vi "MessageTimeOk.vi"(2 "time (ms)":i32=2000, 4 "missage":string) -> ()   [LabVIEW 2015, in "VIPM2.lvlib"]
doc: "Show a message to user in a new window, height dinamicly. Closed by OK button or parametric time (ms)."
uses:
  VIPM2.lvlib
panel:
  in  "Button":bool
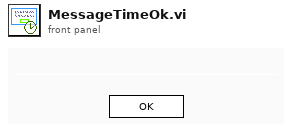
[diagram p1: front panel]
types:
  T1 = typedef "LVRectTypeDef.ctl" = cluster{"Left":i16, "Top":i16, "Right":i16, "Bottom":i16}
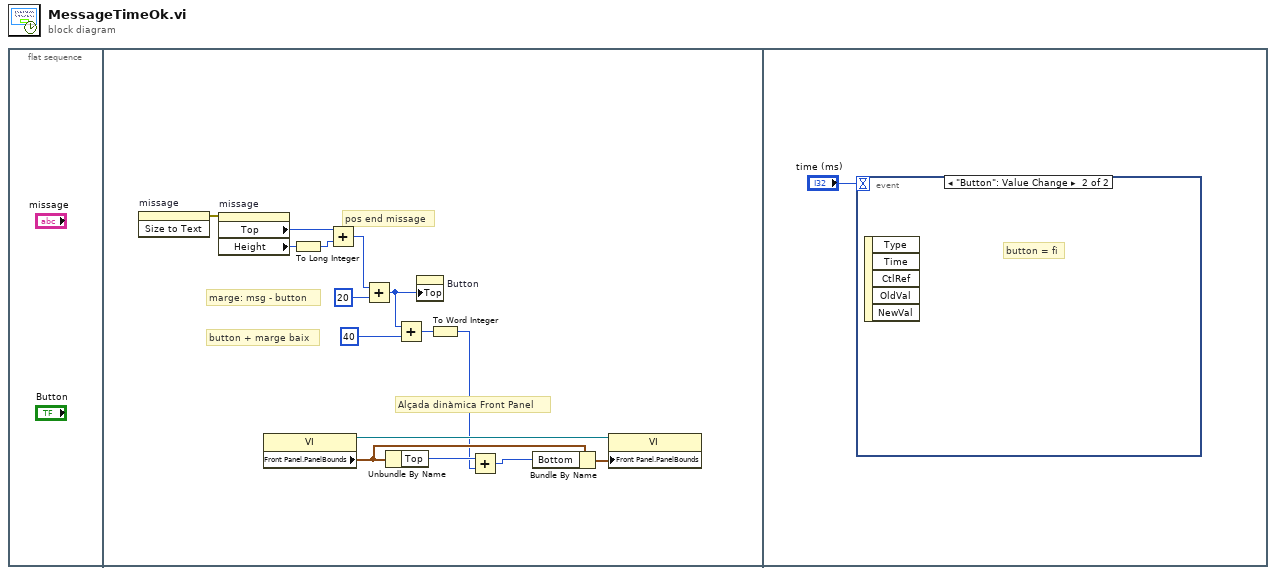
[diagram p0: block diagram]
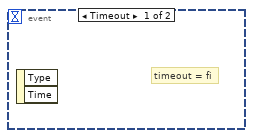
[diagram p2: hidden frame]
diagram:
  n1 = flat-sequence {
    frame #0 {
    }
    frame #1 {
      # "Alçada dinàmica Front Panel"
      # "button + marge baix"
      # "marge: msg - button"
      # "pos end missage"
      n2 = invoke on="missage" class="Str" method="Size to Text"() -> (error out=w5:errorcluster)  [unwired: 3 in, 2 out]
      n3 = property on="missage" class="Str"(error in=w5) -> ("Top"=w15:i32, "Height"=w4:u32)  [unwired: 1 in, 2 out]
      n4 = property class="VI"() -> (reference out=w12:refnum<vi>, "Front Panel.PanelBounds"=w11:T1)  [unwired: 2 in, 1 out]
      n5 = To Long Integer(number=w4) -> (32bit integer=w3:i32)
      n6 = Add(x=w15, y=w3) -> (x+y=w14:i32)
      n7 = Add(x=w14, y=20) -> (x+y=w13:i32)
      n8 = Unbundle By Name(w11) -> ("Top"=w9:i16)
      n9 = Add(x=w13, y=40) -> (x+y=w2:i32)
      n10 = property on="Button" class="Bool"("Top"=w13) -> ()  [unwired: 2 in, 2 out]
      n11 = To Word Integer(number=w2) -> (16bit integer=w1:i16)
      n12 = Add(x=w9, y=w1) -> (x+y=w8:i16)
      n13 = Bundle By Name(cluster=w11, "Bottom"=w8) -> (w10:T1)
      n14 = property class="VI"(reference=w12, "Front Panel.PanelBounds"=w10) -> ()  [unwired: 1 in, 2 out]
    }
    frame #2 {
      n15 = event shown="[1] \"Button\": Value Change" {
        selector: _ -> [_ _]
        dyn-events: _ -> [_ _]
        timeout: "time (ms)" -> [_ _]
        event Timeout {
          # "timeout = fi"
          n16 = event-data() -> ()  [unwired: 1 in, 2 out]
        }
        event "Button": Value Change {
          # "button = fi"
          n17 = event-data() -> ()  [unwired: 1 in, 5 out]
        }
      }
    }
  }
